vi "regulation2.vi"(8 "error in (no error)":errorcluster, 10 "fmin":dbl, 11 "fmax":dbl) -> (0 "error out":errorcluster)   [LabVIEW 2015, in "SCANalone4x64.lvlib"]
doc: "__declspec(dllimport) void __stdcall regulation2(double fmax, double fmin);"
uses:
  <userlib>/SCANalone4x64/SCANalone4x64.lvlib
  <userlib>/SCANalone4x64/SCANalone4x64.dll
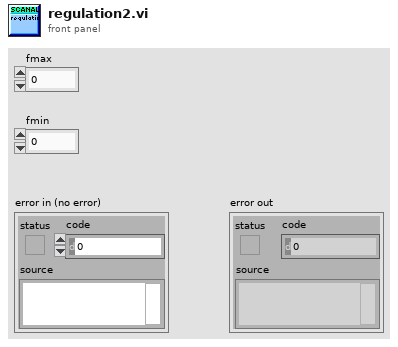
[diagram p1: front panel]
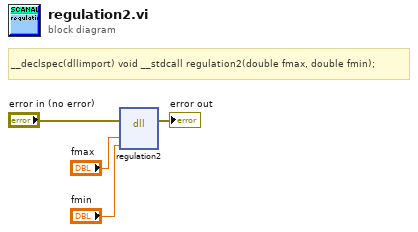
[diagram p0: block diagram]
diagram:
  # "__declspec(dllimport) void __stdcall regulation2(double fmax, double fmin);"
  n1 = dll-call lib="C:/Program Files/National Instruments/LabVIEW 2015/user.lib/SCANalone4x64/SCANalone4x64.*" fn="regulation2"(error in="error in (no error)", "fmax"="fmax", "fmin"="fmin") -> (error out=→"error out":errorcluster)  [unwired: 5 in, 1 out]
